vi "Convert-U32-Array-to-U8-Array.vi"(11 "state":u32[](array[numeric]) format="%.0x") -> (3 "Array":u8[](array[numeric]) format="%.0x")   [LabVIEW 2017]
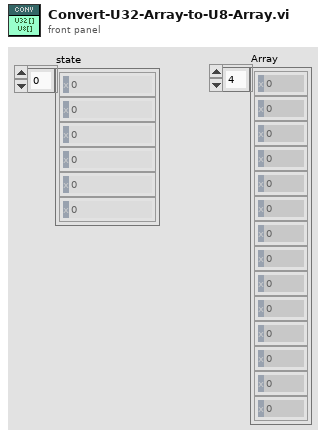
[diagram p1: front panel]
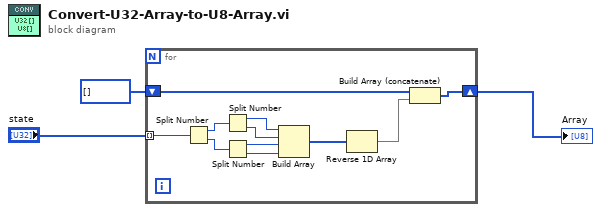
[diagram p0: block diagram]
diagram:
  n1 = for {
    shift-right: [w6] -> w3
    shift-left: u8[] [] -> [w11]
    tunnel: "state" -> [w14] mode=indexing
    n2 = Split Number(x=w14) -> (hi(x)=w12:u16, lo(x)=w13:u16)
    n3 = Split Number(x=w12) -> (hi(x)=w7:u8, lo(x)=w8:u8)
    n4 = Split Number(x=w13) -> (hi(x)=w9:u8, lo(x)=w10:u8)
    n5 = Build Array(w7, w8, w9, w10) -> (w5:u8[])
    n6 = Reverse 1D Array(array=w5) -> (reversed array=w4:u8[])
    n7 = Build Array (concatenate)(w11, w4) -> (w6:u8[])
  }
  "Array" <- w3
